vi "Actor Core.vi"(8 "error in":errorcluster, 11 "Nested in":refnum<class "Valve.lvclass">) -> (0 "error out":errorcluster, 3 "Actor out":refnum<class "Actor.lvclass">)   [LabVIEW 2021, in "Valve.lvlib" / "Valve.lvclass"]
doc: "(<B>Filename</B>: Actor Framework.lvlib:Actor.lvclass:Actor Core.vi)\n\nReceives messages to the actor, reacts to them, and initiates any error handling that may shut the actor down.\n\nDescendant classes may override this VI to append parallel tasks for the actor to complete while it handles messages. Overrides use the Call Parent Method node."
uses:
  Valve.lvclass
  Valve.lvclass/Valve.ctl
  <vilib>/ActorFramework/Actor/Actor.lvclass
  <vilib>/ActorFramework/Stop Msg/Stop Msg.lvclass
  <vilib>/MGI/Panel Manager/Panel Actor/Panel Actor/Panel Actor.lvclass
  Valve Messages/Update State Msg/Update State Msg.lvclass
  C:/Program Files/National Instruments/LabVIEW 2021/vi.lib/MGI/Panel Manager/Panel Actor/Panel Actor/Panel Actor.lvclass
  C:/Program Files/National Instruments/LabVIEW 2021/vi.lib/ActorFramework/Actor/Actor.lvclass
  C:/PPLs/Valve/Valve/Valve.lvclass
panel:
  in  "Open?":bool
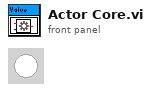
[diagram p1: front panel]
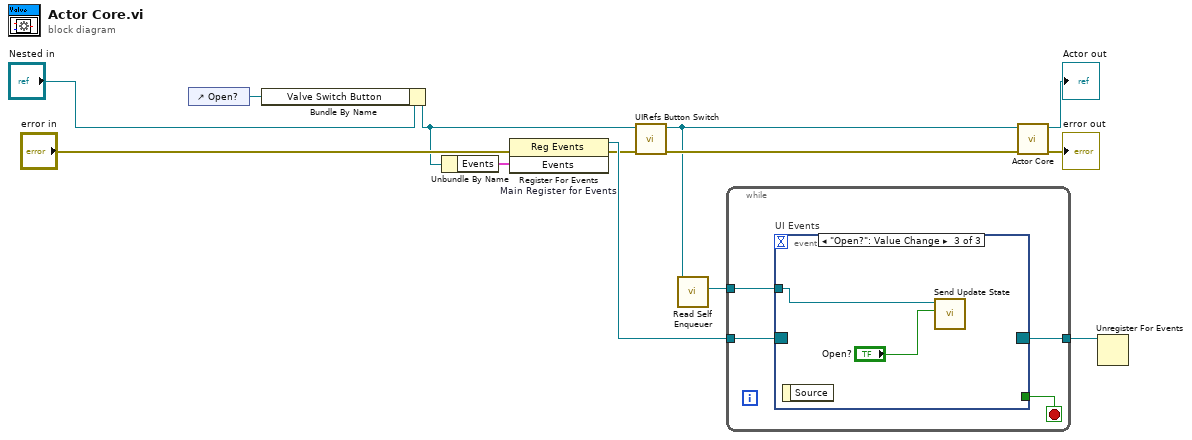
[diagram p0: block diagram]
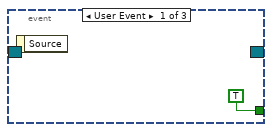
[diagram p2: hidden frame]
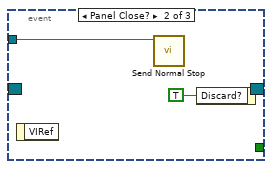
[diagram p3: hidden frame]
diagram:
  n1 = control-ref of="Open?"() -> (w2:refnum<vi>)
  n2 = Bundle By Name(cluster="Nested in", "Valve Switch Button"=w2) -> (w3:refnum<class "Valve.lvclass">)
  n3 = Unbundle By Name(w3) -> ("Events"=w10:cluster{"Stop":refnum<user-event>})
  n4 = register-events "Main Register for Events"(error in="error in", w10) -> (reference out=w11:refnum<event-registration>, error out=w6:errorcluster)  [unwired: 1 in]
  n5 = call "UIRefs Button Switch.vi"("error in (no error)"=w6, "Valve in"=w3) -> ("error out"=w5:errorcluster, "Valve out"=w1:refnum<class "Valve.lvclass">)  [unwired: 8 in]
  n6 = call <vilib>:"Read Self Enqueuer.vi"("Actor"=w1) -> ("Self Enqueuer"=w8:refnum<class "Message Enqueuer.lvclass">)  [unwired: 10 in]
  n7 = while {
    tunnel: w11 -> [w17]
    tunnel: [w15] -> w9
    tunnel: w8 -> [w14]
    stop <- w16 stop-if-true
    n8 = event "UI Events" shown="[2] \"Open?\": Value Change" {
      selector: w17 -> [_ _ _]
      dyn-events: [_ _ _] -> w15
      timeout: _ -> [_ _ _]
      tunnel: [TRUE _ _] -> w16
      tunnel: w14 -> [_ w19 w22]
      event User Event {
        n9 = event-data() -> ()  [unwired: 1 in, 1 out]
      }
      event Panel Close? {
        n10 = event-data() -> ()  [unwired: 1 in, 1 out]
        n11 = call <vilib>:"Send Normal Stop.vi"("Message Enqueuer"=w19) -> ()  [unwired: 10 in, 1 out]
        n12 = event-data("Discard?"=TRUE) -> ()  [unwired: 1 in, 1 out]
      }
      event "Open?": Value Change {
        n13 = event-data() -> ()  [unwired: 1 in, 1 out]
        n14 = call "Send Update State.vi"("Open?"="Open?", "Message Enqueuer"=w22) -> ()  [unwired: 8 in, 2 out]
      }
    }
  }
  n15 = call-parent "Actor Core.vi"("error in"=w5, "Panel Actor in"=w1) -> ("error out"=→"error out":errorcluster, "Actor out"=→"Actor out":refnum<class "Actor.lvclass">)  [unwired: 8 in]
  n16 = Unregister For Events(event registration refnum=w9) -> ()  [unwired: 1 in, 1 out]
